vi "Initialize Server.vi"(8 "error in (no error)":errorcluster, 11 "Base Server in":refnum<class "Server.lvclass">) -> (0 "error out":errorcluster, 3 "Base Server out":refnum<class "Server.lvclass">)   [LabVIEW 2024, in "Ramses Framework.lvlib" / "Server.lvclass"]
uses:
  Server.lvclass
  Service/Service.lvclass
  Server.lvclass/Server.ctl
  Write Server Running.vi
  Loop.vi
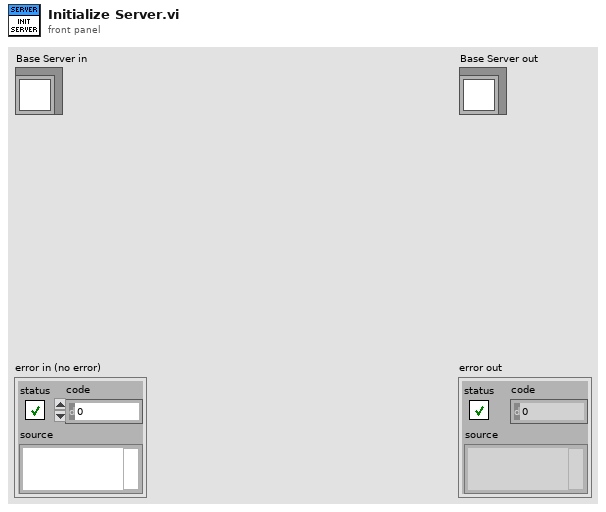
[diagram p1: front panel]
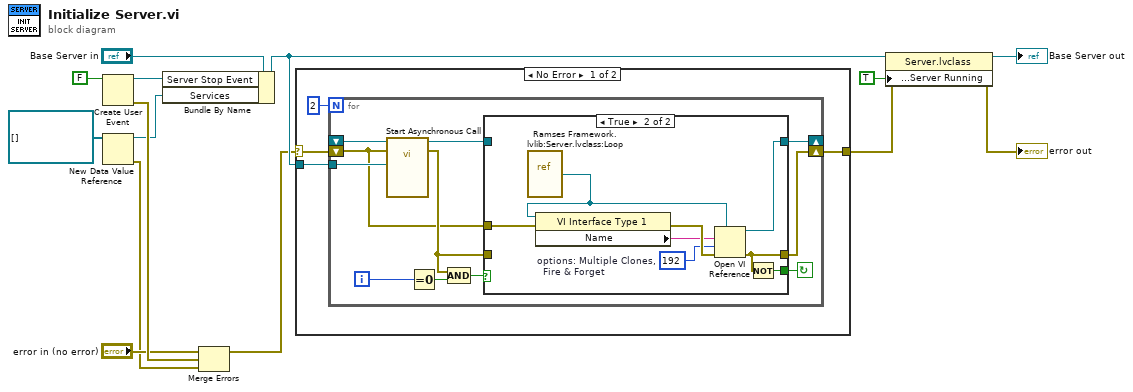
[diagram p0: block diagram]
diagram:
  n1 = Create User Event(user event datatype=FALSE ("Stop")) -> (user event=w8:refnum<user-event>, error out=w14:errorcluster)  [unwired: 1 in]
  n2 = New Data Value Reference(data value=refnum<class "Service.lvclass">[] [] ("Services")) -> (data value reference=w7:refnum<data-value>, error out=w6:errorcluster)  [unwired: 1 in]
  n3 = Bundle By Name(cluster="Base Server in", "Server Stop Event"=w8, "Services"=w7) -> (w10:refnum<class "Server.lvclass">)
  n4 = Merge Errors("error in (no error)", w14, w6) -> (w2:errorcluster)
  n5 = case shown="No Error" w2 {
    selector: w2 -> [w15 w40]
    tunnel: w10 -> [w18 _]
    tunnel: [w16 w40] -> w1
    frame No Error {
      n6 = for {
        N: 2 -> [_]
        tunnel: w18 -> [w29]
        shift-right: [w28] -> _
        shift-left: _ -> [w27]
        shift-right: [w25] -> w16
        shift-left: w15 -> [w19]
        i -> [w22]
        stop <- w20 continue-if-true
        n7 = call-by-ref "Start Asynchronous Call"(reference=w27, error in=w19, "Base Server in"=w29) -> (reference out=w26:refnum<vi>, error out=w21:errorcluster)  [unwired: 11 in]
        n8 = Equal To 0?(x=w22) -> (x = 0?=w23:bool)
        n9 = Compound Arithmetic op=AND(w21, w23) -> (w24:bool)
        n10 = case shown="True" w24 {
          tunnel: [w31 w36] -> w28
          tunnel: [w30 w34] -> w25
          tunnel: w26 -> [w31 _]
          tunnel: w21 -> [w30 _]
          tunnel: [_ w35] -> w20
          tunnel: w19 -> [_ w33]
          frame False {
          }
          frame True {
            w37 = 192  # options: Multiple Clones,   Fire & Forget
            n11 = vi-ref "Ramses Framework.lvlib:Server.lvclass:Loop.vi"() -> (w32:refnum<vi>)
            n12 = property class="VI Interface Type 1"(reference=w32, error in=w33) -> (error out=w39:errorcluster, "Name"=w38:string)  [unwired: 1 out]
            n13 = Open VI Reference(type specifier VI Refnum (for type only)=w32, vi path=w38, options=w37, error in (no error)=w39) -> (vi reference=w36:refnum<vi>, error out=w34:errorcluster)  [unwired: 2 in]
            n14 = Not(x=w34) -> (.not. x?=w35:bool)
          }
        }
      }
    }
    frame Error {
    }
  }
  n15 = property class="Server.lvclass"(reference=w10, error in=w1, "Public API:Accessors:Server Running"=TRUE ("Server Running")) -> (reference out=→"Base Server out":refnum<class "Server.lvclass">, error out=→"error out":errorcluster)
